vi "iRobot UART Write.vi"(8 "error in":errorcluster, 9 "data":u8[](array[numeric]), 11 "UART port in":T1) -> (0 "error out":errorcluster, 3 "UART port out":T1)   [LabVIEW 2015]
doc: "Write data to the UART transmit buffer."
uses:
  iRobot UART Port Type.ctl
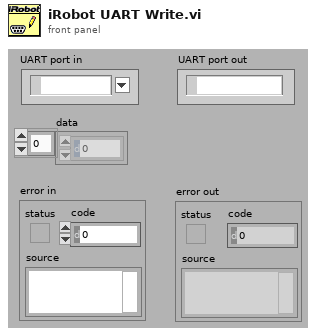
[diagram p1: front panel]
types:
  T1 = typedef "iRobot UART Port Type.ctl" = refnum<visa-resource-name>
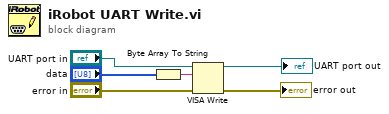
[diagram p0: block diagram]
diagram:
  n1 = Byte Array To String(unsigned byte array="data") -> (string=w1:string)
  n2 = VISA Write(VISA resource name="UART port in", write buffer=w1, error in (no error)="error in") -> (VISA resource name out=→"UART port out":T1, error out=→"error out":errorcluster)  [unwired: 1 out]
